vi "MSScript_SubVI_NonCMNTIndexRecovery.vi"(5 "SEL of CMNT":cluster{"Start":u32, "End":u32}[](array[cluster]), 6 "NonCMNT.SEL":cluster{"Start":u32, "End":u32}[](array[cluster])) -> (1 "RecoverySEL":cluster{"Start":u32, "End":u32}[](array[cluster]))   [LabVIEW 2018, in "MSScript.lvclass"]
uses:
  MSScript.lvclass
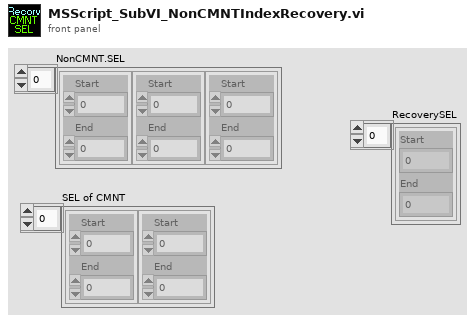
[diagram p1: front panel]
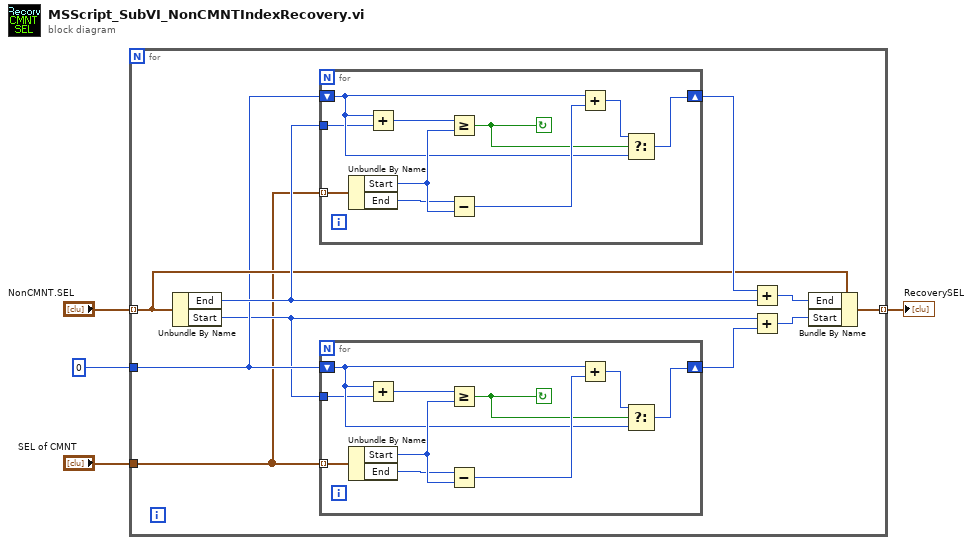
[diagram p0: block diagram]
diagram:
  n1 = for {
    tunnel: "SEL of CMNT" -> [w6]
    tunnel: "NonCMNT.SEL" -> [w9] mode=indexing
    tunnel: [w14] -> w2 mode=indexing
    tunnel: u32 0 -> [w8]
    n2 = Unbundle By Name(w9) -> ("End"=w10:u32, "Start"=w7:u32)
    n3 = for {
      tunnel: w6 -> [w34] mode=indexing
      shift-right: [w31] -> w13
      shift-left: w8 -> [w27]
      tunnel: w10 -> [w25]
      stop <- w30 continue-if-true
      n4 = Unbundle By Name(w34) -> ("Start"=w29:u32, "End"=w28:u32)
      n5 = Add(x=w27, y=w25) -> (x+y=w26:u32)
      n6 = Greater Or Equal?(x=w26, y=w29) -> (x >= y?=w30:bool)
      n7 = Subtract(x=w28, y=w29) -> (x-y=w33:u32)
      n8 = Add(x=w27, y=w33) -> (x+y=w32:u32)
      n9 = Select(t=w32, s=w30, f=w27) -> (s? t:f=w31:u32)
    }
    n10 = for {
      tunnel: w6 -> [w24] mode=indexing
      shift-right: [w21] -> w5
      shift-left: w8 -> [w17]
      tunnel: w7 -> [w15]
      stop <- w20 continue-if-true
      n11 = Unbundle By Name(w24) -> ("Start"=w19:u32, "End"=w18:u32)
      n12 = Add(x=w17, y=w15) -> (x+y=w16:u32)
      n13 = Greater Or Equal?(x=w16, y=w19) -> (x >= y?=w20:bool)
      n14 = Subtract(x=w18, y=w19) -> (x-y=w23:u32)
      n15 = Add(x=w17, y=w23) -> (x+y=w22:u32)
      n16 = Select(t=w22, s=w20, f=w17) -> (s? t:f=w21:u32)
    }
    n17 = Add(x=w13, y=w10) -> (x+y=w11:u32)
    n18 = Add(x=w7, y=w5) -> (x+y=w12:u32)
    n19 = Bundle By Name(cluster=w9, "End"=w11, "Start"=w12) -> (w14:cluster{"Start":u32, "End":u32})
  }
  "RecoverySEL" <- w2
